vi "State_Machine.vi"(8 "error in (no error)":errorcluster caption="entrée d'erreur (pas d'erreur)", 11 "Stop_Ana IN":refnum<class "Stop_Ana.lvclass">) -> (0 "error out":errorcluster caption="sortie d'erreur", 2 "Json_String":string, 3 "Stop_Ana Out":refnum<class "Stop_Ana.lvclass">)   [LabVIEW 2020, in "Library Test.lvlib" / "Stop_Ana.lvclass"]
uses:
  Stop_Ana.lvclass
  C:/Users/ngarcin/OneDrive - Altyor/Standard TB/Suite TB45/Class/Test/Test (Default)/Test (Default).lvclass
  Commun VI/TypeDef/Variable Printable.ctl
  7f5f09f5-24fc-40b2-86d1-babc68c912a0.vi
  Instrument/Instrument (Default)/Class Instrument (Default).lvclass
  Commun VI/Library Commun.lvlib
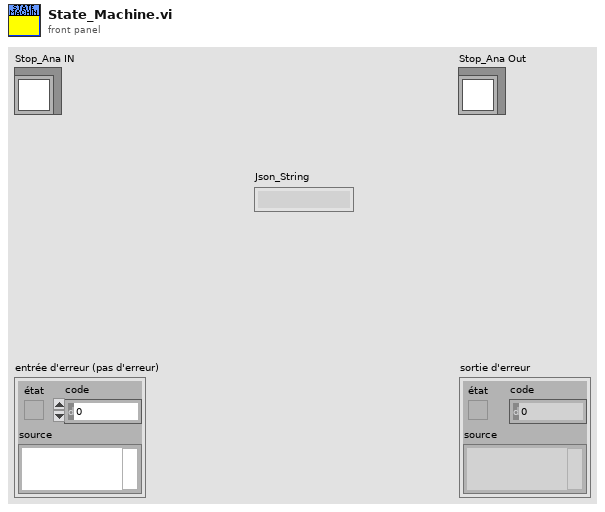
[diagram p1: front panel]
types:
  T1 = typedef "Variable Printable.ctl" = string
  T2 = enum16{"Get Variable", "Get All Variables", "Set Variable", "Delete Variable", "Delete All Variable"}
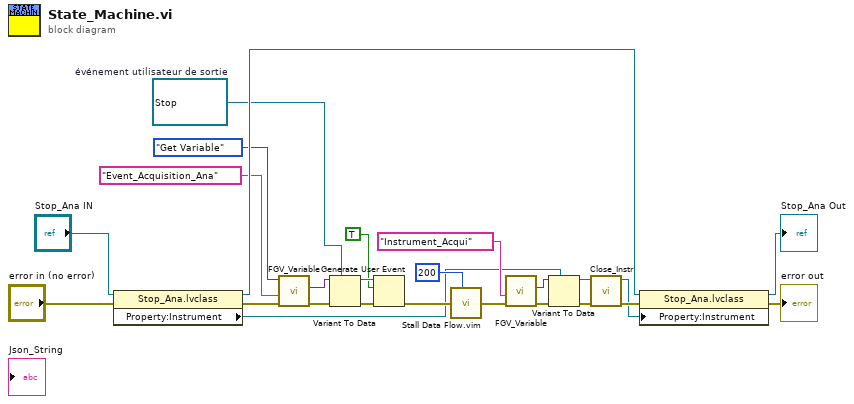
[diagram p0: block diagram]
diagram:
  w16 = refnum<user-event> refnum  # événement utilisateur de sortie
  n1 = property class="Stop_Ana.lvclass"(reference="Stop_Ana IN", error in="error in (no error)") -> (reference out=w24:refnum<class "Stop_Ana.lvclass">, error out=w15:errorcluster, "Property:Instrument"=w2:refnum<class "Class Instrument (Default).lvclass">)
  n2 = call "FGV_Variable.vi"("error in (no error)"=w15, "Variable"=T1 "Event_Acquisition_Ana", "Function"=T2."Get Variable") -> ("error out"=w18:errorcluster, "Data Out"=w17:variant)  [unwired: 6 in, 1 out]
  n3 = Variant To Data(error in=w18, type=w16, Variant=w17) -> (data=w12:refnum<user-event>, error out=w11:errorcluster)
  n4 = Generate User Event(user event=w12, event data cluster=TRUE ("données d'événement"), error in=w11) -> (error out=w10:errorcluster)  [unwired: 1 in, 1 out]
  n5 = call "Stall Data Flow.vim"("value in"=w10, "milliseconds to wait"=u32 200) -> ("value out"=w6:errorcluster)  [unwired: 1 out]
  n6 = call "FGV_Variable.vi"("error in (no error)"=w6, "Variable"=T1 "Instrument_Acqui") -> ("error out"=w5:errorcluster, "Data Out"=w3:variant)  [unwired: 7 in, 1 out]
  n7 = Variant To Data(error in=w5, type=w2, Variant=w3) -> (data=w1:refnum<class "Class Instrument (Default).lvclass">, error out=w4:errorcluster)
  n8 = call-dynamic "Close_Instr.vi"("error in (no error)"=w4, "Class Instrument (Default) en entrée"=w1) -> ("error out"=w14:errorcluster, "Class Instrument (Default) en sortie"=w13:refnum<class "Class Instrument (Default).lvclass">)  [unwired: 8 in]
  n9 = property class="Stop_Ana.lvclass"(reference=w24, error in=w14, "Property:Instrument"=w13) -> (reference out=→"Stop_Ana Out":refnum<class "Stop_Ana.lvclass">, error out=→"error out":errorcluster)
